vi "FCI Lip Symmetry.vi"(0 "Calibrated Image":T1, 5 "Box All Edges":T3, 7 "Lip Outer Perpendicular lines":T2(array[cluster]), 9 "Image in":T1(plugin-control), 11 "error in (no error)":errorcluster) -> (6 "Lip symmetry":dbl, 15 "error out":errorcluster)   [LabVIEW 2019, in "Algorithm.lvclass"]
uses:
  FrameworkOverrides/Algorithm.lvclass
  <vilib>/vision/NI_Vision_Development_Module.lvlib
  <vilib>/vision/Image Controls.llb/IMAQ Image.ctl
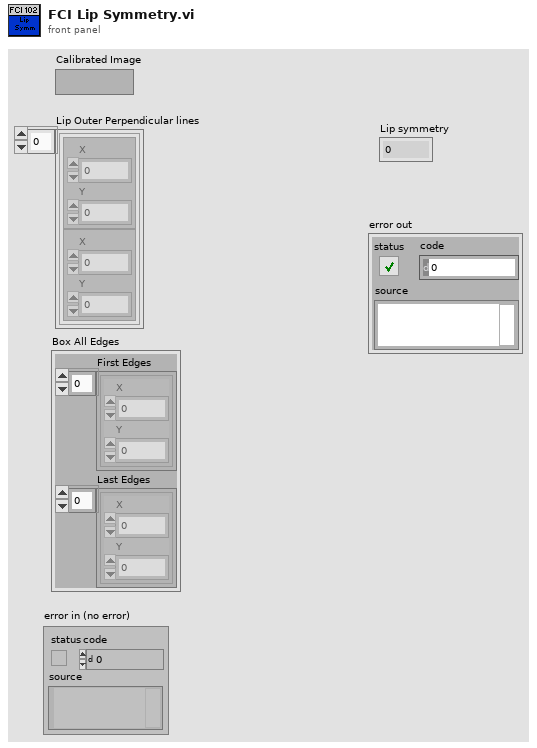
[diagram p1: front panel]
types:
  T1 = typedef "IMAQ Image.ctl" = refnum<image>
  T2 = cluster{cluster{"X":sgl, "Y":sgl}, cluster{"X":sgl, "Y":sgl}}[]
  T3 = cluster{"First Edges":cluster{"X":sgl, "Y":sgl}[], "Last Edges":cluster{"X":sgl, "Y":sgl}[]}
  T4 = cluster{"Point 1":cluster{"X":sgl, "Y":sgl}, "Point 2":cluster{"X":sgl, "Y":sgl}}
  T5 = cluster{cluster{"X":sgl, "Y":sgl}, cluster{"X":sgl, "Y":sgl}}
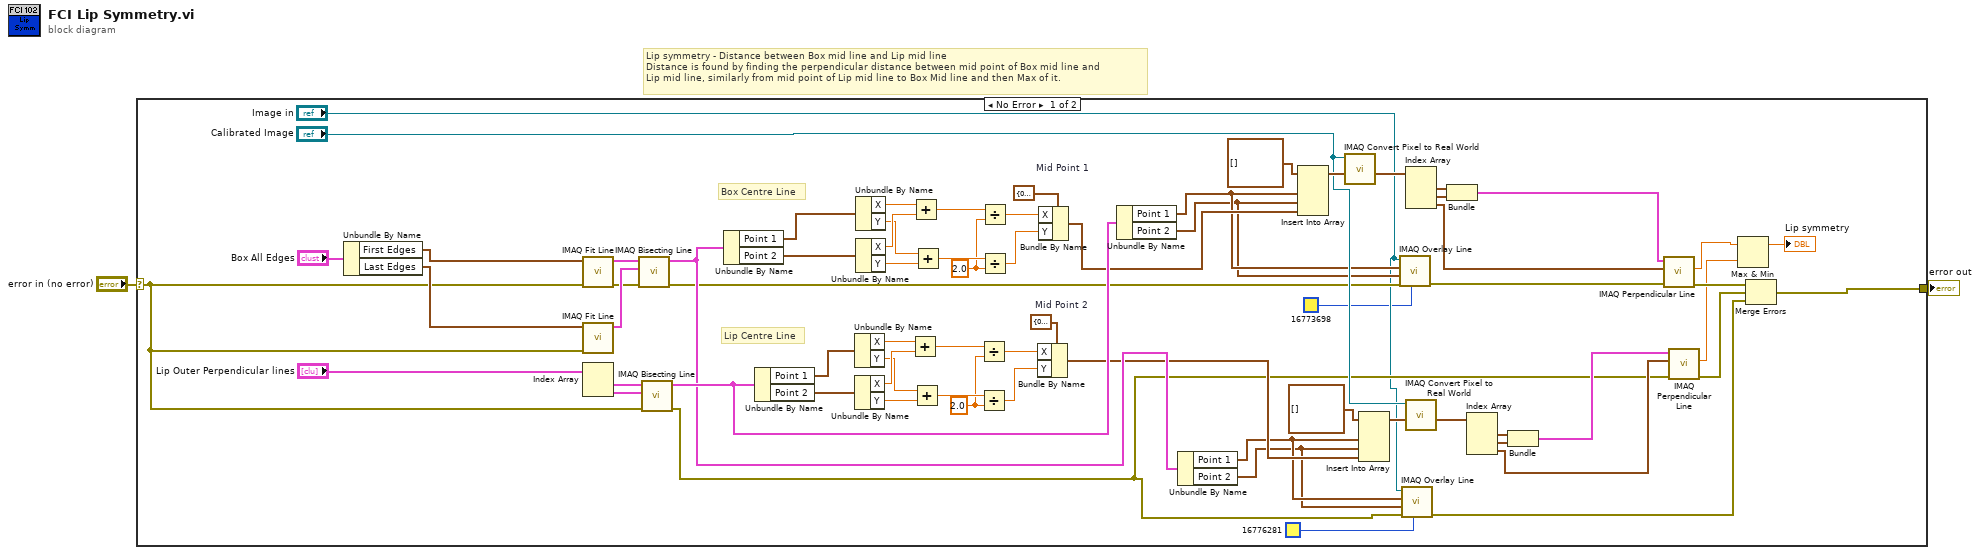
[diagram p0: block diagram]
diagram:
  # "Lip symmetry - Distance between Box mid line and Lip mid line\nDistance is found by finding the perpendicular distance between mid point of Box mid line and\nLip mid line, similarly from mid point of Lip mid line to Box Mid line and then Max of it."
  n1 = case shown="No Error" "error in (no error)" {
    selector: "error in (no error)" -> [w38 w73]
    tunnel: [w39 w73] -> w1
    frame No Error {
      w45 = sgl 2.0 ("y")
      w55 = sgl 2.0 ("y")
      # "Lip Centre Line"
      # "Box Centre Line"
      n2 = Unbundle By Name("Box All Edges") -> ("First Edges"=w72:cluster{"X":sgl, "Y":sgl}[], "Last Edges"=w71:cluster{"X":sgl, "Y":sgl}[])
      n3 = call "IMAQ Fit Line"("error in (no error)"=w38, "Points"=w72) -> ("error out"=w66:errorcluster, "Line Segment"=w70:T4)  [unwired: 4 in, 4 out]
      n4 = call "IMAQ Fit Line"("error in (no error)"=w38, "Points"=w71) -> ("Line Segment"=w69:T4)  [unwired: 4 in, 5 out]
      n5 = Index Array(array="Lip Outer Perpendicular lines") -> (element #1=w65:T5, element #2=w64:T5)  [unwired: 2 in]
      n6 = call "IMAQ Bisecting Line"("error in (no error)"=w66, "Line 2"=w69, "Line 1"=w70) -> ("error out"=w8:errorcluster, "Bisecting Line"=w18:T4)  [unwired: 7 in]
      n7 = call "IMAQ Bisecting Line"("error in (no error)"=w38, "Line 2"=w64, "Line 1"=w65) -> ("error out"=w9:errorcluster, "Bisecting Line"=w32:T4)  [unwired: 7 in]
      n8 = Unbundle By Name(w18) -> ("Point 1"=w63:cluster{"X":sgl, "Y":sgl}, "Point 2"=w62:cluster{"X":sgl, "Y":sgl})
      n9 = Unbundle By Name(w32) -> ("Point 1"=w41:cluster{"X":sgl, "Y":sgl}, "Point 2"=w40:cluster{"X":sgl, "Y":sgl})
      n10 = Unbundle By Name(w41) -> ("X"=w51:sgl, "Y"=w49:sgl)
      n11 = Unbundle By Name(w40) -> ("X"=w50:sgl, "Y"=w48:sgl)
      n12 = Unbundle By Name(w63) -> ("X"=w61:sgl, "Y"=w59:sgl)
      n13 = Unbundle By Name(w62) -> ("X"=w60:sgl, "Y"=w58:sgl)
      n14 = Add(x=w51, y=w50) -> (x+y=w47:sgl)
      n15 = Add(x=w61, y=w60) -> (x+y=w57:sgl)
      n16 = Add(x=w49, y=w48) -> (x+y=w46:sgl)
      n17 = Add(x=w59, y=w58) -> (x+y=w56:sgl)
      n18 = Divide(x=w47, y=w45) -> (x/y=w43:sgl)
      n19 = Divide(x=w46, y=w45) -> (x/y=w42:sgl)
      n20 = Divide(x=w57, y=w55) -> (x/y=w53:sgl)
      n21 = Divide(x=w56, y=w55) -> (x/y=w52:sgl)
      n22 = Bundle By Name "Mid Point 2"(cluster=cluster{"X":sgl, "Y":sgl} {"X"=0.0, "Y"=0.0} ("Point 1"), "X"=w43, "Y"=w42) -> (w16:cluster{"X":sgl, "Y":sgl})
      n23 = Bundle By Name "Mid Point 1"(cluster=cluster{"X":sgl, "Y":sgl} {"X"=0.0, "Y"=0.0} ("Point 1"), "X"=w53, "Y"=w52) -> (w25:cluster{"X":sgl, "Y":sgl})
      n24 = Unbundle By Name(w32) -> ("Point 1"=w13:cluster{"X":sgl, "Y":sgl}, "Point 2"=w12:cluster{"X":sgl, "Y":sgl})
      n25 = Unbundle By Name(w18) -> ("Point 1"=w11:cluster{"X":sgl, "Y":sgl}, "Point 2"=w10:cluster{"X":sgl, "Y":sgl})
      n26 = Insert Into Array(array=cluster{"X":sgl, "Y":sgl}[] [] ("appended array"), new element #1=w13, new element #2=w12, new element #3=w25) -> (w30:cluster{"X":sgl, "Y":sgl}[])  [unwired: 1 in]
      n27 = call "IMAQ Convert Pixel to Real World"("Array of Pixel Coordinates"=w30, "Calibrated Image"="Calibrated Image") -> ("Array of Real World Coordinates"=w29:cluster{"X":sgl, "Y":sgl}[])  [unwired: 4 in, 5 out]
      n28 = Insert Into Array(array=cluster{"X":sgl, "Y":sgl}[] [] ("appended array"), new element #1=w11, new element #2=w10, new element #3=w16) -> (w22:cluster{"X":sgl, "Y":sgl}[])  [unwired: 1 in]
      n29 = call "IMAQ Overlay Line"("Color"=u32 16773698, "error in (no error)"=w8, "End Point"=w12, "Start Point"=w13, "Image"="Image in") -> ("error out"=w7:errorcluster)  [unwired: 5 in, 1 out]
      n30 = call "IMAQ Overlay Line"("Color"=u32 16776281, "error in (no error)"=w9, "End Point"=w10, "Start Point"=w11, "Image"="Image in") -> ("error out"=w6:errorcluster)  [unwired: 5 in, 1 out]
      n31 = Index Array(array=w29) -> (element #1=w28:cluster{"X":sgl, "Y":sgl}, element #2=w27:cluster{"X":sgl, "Y":sgl}, element #3=w24:cluster{"X":sgl, "Y":sgl})  [unwired: 3 in]
      n32 = call "IMAQ Convert Pixel to Real World"("Array of Pixel Coordinates"=w22, "Calibrated Image"="Calibrated Image") -> ("Array of Real World Coordinates"=w21:cluster{"X":sgl, "Y":sgl}[])  [unwired: 4 in, 5 out]
      n33 = Bundle(w28, w27) -> (w26:T5)  [unwired: 1 in]
      n34 = Index Array(array=w21) -> (element #1=w20:cluster{"X":sgl, "Y":sgl}, element #2=w19:cluster{"X":sgl, "Y":sgl}, element #3=w15:cluster{"X":sgl, "Y":sgl})  [unwired: 3 in]
      n35 = Bundle(w20, w19) -> (w17:T5)  [unwired: 1 in]
      n36 = call "IMAQ Perpendicular Line"("error in (no error)"=w7, "Point"=w24, "Line"=w26) -> ("error out"=w37:errorcluster, "Distance"=w35:dbl)  [unwired: 6 in, 1 out]
      n37 = call "IMAQ Perpendicular Line"("error in (no error)"=w9, "Point"=w15, "Line"=w17) -> ("error out"=w33:errorcluster, "Distance"=w34:dbl)  [unwired: 6 in, 1 out]
      n38 = Max & Min(x=w35, y=w34) -> (max(x,y)=→"Lip symmetry":dbl)  [unwired: 1 out]
      n39 = Merge Errors(w37, w33, w6) -> (w39:errorcluster)
    }
    frame Error {
    }
  }
  "error out" <- w1
